vi "Autonomous Independent.vi"() -> ()   [LabVIEW 2016]
doc: "This VI is called when autonomous begins, and will automatically be terminated when autonomous ends. You can carry out timed or sensor driven robot movement independently without needing to return to the caller."
uses:
  <vilib>/Rock Robotics/WPI/ThirdParty/CanMotor/CTRLib-LV-TalonSRX/Framework/ServoParams.ctl
  <vilib>/Rock Robotics/WPI/ThirdParty/CanMotor/CTRLib-LV-TalonSRX/CTRE_CANTalonSRX_ControlMode.ctl
  <vilib>/Rock Robotics/WPI/Utilities/WPI_GetSetVariantRefNum.vi
  <vilib>/Rock Robotics/Network Tables/NT Write Numeric Array.vi
  <vilib>/Rock Robotics/WPI/ThirdParty/CanMotor/CTRLib-LV-TalonSRX/Framework/CTRE_ServoBlock_SmartTankStraightDistanceImu.vi
  <vilib>/Rock Robotics/WPI/ThirdParty/CanMotor/CTRLib-LV-TalonSRX/Framework/CTRE_ServoBlock_SmartTankTurnImu.vi
  <vilib>/Rock Robotics/WPI/ThirdParty/CanMotor/CTRLib-LV-TalonSRX/Framework/CTRE_ServoBlock_SmartTank.vi
panel:
  in  "Distance Params Back Up":T1={"P"=0.049999999999999996, "I"=0.001, "D"=0.017000000000000005, "I-Accum Max"=0.1, "I-Zone"=2.0, "Max Output"=0.5, "Nominal Output"=0.0, "Allowable Error"=0.0, "Reset I Accum"=FALSE}
  in  "Straight Params Back Up":T1={"P"=0.03, "I"=0.002, "D"=0.0, "I-Accum Max"=0.07, "I-Zone"=1.0, "Max Output"=0.15, "Nominal Output"=0.0, "Allowable Error"=0.5, "Reset I Accum"=FALSE}
  in  "Distance Params To Peg":T1={"P"=0.049999999999999996, "I"=0.001, "D"=0.017000000000000005, "I-Accum Max"=0.1, "I-Zone"=2.0, "Max Output"=0.5, "Nominal Output"=0.0, "Allowable Error"=0.0, "Reset I Accum"=FALSE}
  in  "Straight Params To Peg":T1={"P"=0.03, "I"=0.002, "D"=0.0, "I-Accum Max"=0.07, "I-Zone"=1.0, "Max Output"=0.15, "Nominal Output"=0.0, "Allowable Error"=0.5, "Reset I Accum"=FALSE}
  in  "Turn To Airship":T1={"P"=0.05, "I"=0.004, "D"=0.003, "I-Accum Max"=1.0, "I-Zone"=4.0, "Max Output"=0.2, "Nominal Output"=0.0, "Allowable Error"=0.0, "Reset I Accum"=FALSE}
  in  "Distance Params To Airship":T1={"P"=0.049999999999999996, "I"=0.001, "D"=0.017000000000000005, "I-Accum Max"=0.1, "I-Zone"=2.0, "Max Output"=0.5, "Nominal Output"=0.0, "Allowable Error"=0.0, "Reset I Accum"=FALSE}
  in  "Straight Params To Airship":T1={"P"=0.03, "I"=0.002, "D"=0.0, "I-Accum Max"=0.07, "I-Zone"=1.0, "Max Output"=0.15, "Nominal Output"=0.0, "Allowable Error"=0.5, "Reset I Accum"=FALSE}
  in  "Back Up\nFrom Peg":dbl=-20.0 format="%#_13g"
  in  "Angle\nTo Airship":dbl=30.0 format="%#_13g"
  in  "Distance\nTo Peg":dbl=55.0
  in  "Distance\nTo Airship":dbl=50.0
  # "Be sure to right-click and choose Data Operations>>Make Current Value default if you want to save the array values with the VI"
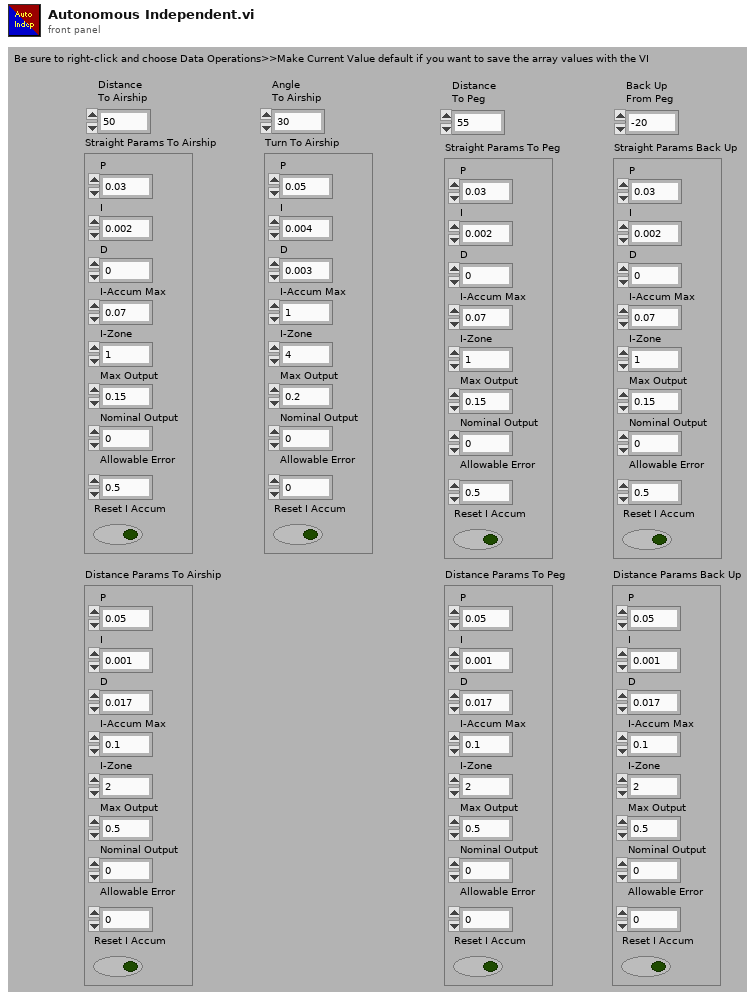
[diagram p1: front panel]
types:
  T1 = typedef "ServoParams.ctl" = cluster{"P":dbl, "I":dbl, "D":dbl, "I-Accum Max":dbl, "I-Zone":dbl, "Max Output":dbl, "Nominal Output":dbl, "Allowable Error":dbl, "Reset I Accum":bool}
  T2 = typedef "WPI_JoystickDevRef.ctl" = cluster{"Device":T3}
  T3 = typedef "WPI_JoystickDeviceEnum.ctl" = enum16{"USB 0", "USB 1", "USB 2", "USB 3", "USB 4", "USB 5"}
  T4 = typedef "SensoredTank.ctl" = cluster{"Sensored Gearbox Left":T5, "Sensored Gearbox Right ":T5, "Wheel Radius":dbl, "Distance Between Wheels":dbl}
  T5 = typedef "SensoredGearbox.ctl" = cluster{"Smart Motor Controller":T6, "Invert":bool, "Gear Ratio":dbl}
  T6 = typedef "WPI_MotorControlDeviceRef.ctl" = cluster{"DeviceStatus":errorcluster, "Type":T7, "PWM":cluster{"PWM Channel":T8, "DeadBand":T9}, "CAN":cluster{"Device Number":u8, "SetOutput VI Ref":variant, "GetOutput VI Ref":variant, "Enable VI Ref":variant, "Disable VI Ref":variant, "Data":variant}, "Invert":bool}
  T7 = typedef "WPI_MotorControlType.ctl" = enum16{"PWM", "CAN"}
  T8 = typedef "FPGA_DIOPWMChannel.ctl" = enum8{"PWM 0", "PWM 1", "PWM 2", "PWM 3", "PWM 4", "PWM 5", "PWM 6", "PWM 7", "PWM 8", "PWM 9", "PWM MXP 0", "PWM MXP 1", "PWM MXP 2", "PWM MXP 3", "PWM MXP 4", "PWM MXP 5", "PWM MXP 6", "PWM MXP 7", "PWM MXP 8", "PWM MXP 9", "Invalid"}
  T9 = typedef "WPI_PWMDeadband.ctl" = cluster{"Name":string, "maxPositivePwm":i32, "minPositivePwm":i32, "centerPwm":i32, "maxNegativePwm":i32, "minNegativePwm":i32, "angularRange":u16}
  T10 = typedef "CTRE_PigeonIMU_DeviceRef.ctl" = cluster{"DeviceStatus":errorcluster, "Device Number":u8, "Type":T11, "Device ID":u32, "Handle":u64, "UsageFrame":u32, "Library Path":path}
  T11 = typedef "CTRE_PigeonIMU_ConnectionType.ctl" = u32
  T12 = typedef "CTRE_CANTalonSRX_ControlMode.ctl" = enum16{"Throttle (Duty-Cycle)", "Position Closed-Loop", "Velocity Closed-Loop", "Current Closed-Loop", "Voltage Compensation", "Slave Follower", "Motion Profile", "Motion Magic"}
  T13 = cluster{"Sensored Tank":T4, "PigeonIMU":T10, "Talon SRX Control Mode":T12, "Set Heading":dbl, "Distance":dbl, "Distance Tolerance":dbl, "Straight Params":T1, "Distance Params":T1}
  T14 = cluster{"Servo Params":T1, "Sensored Tank":T4, "PigeonIMU":T10, "Talon SRX Control Mode":T12, "Angle Tolerance":dbl, "Set Angle":dbl}
  T15 = cluster{"Sensored Tank":T4, "Talon SRX Control Mode":T12, "Forward":dbl, "Turn":dbl}
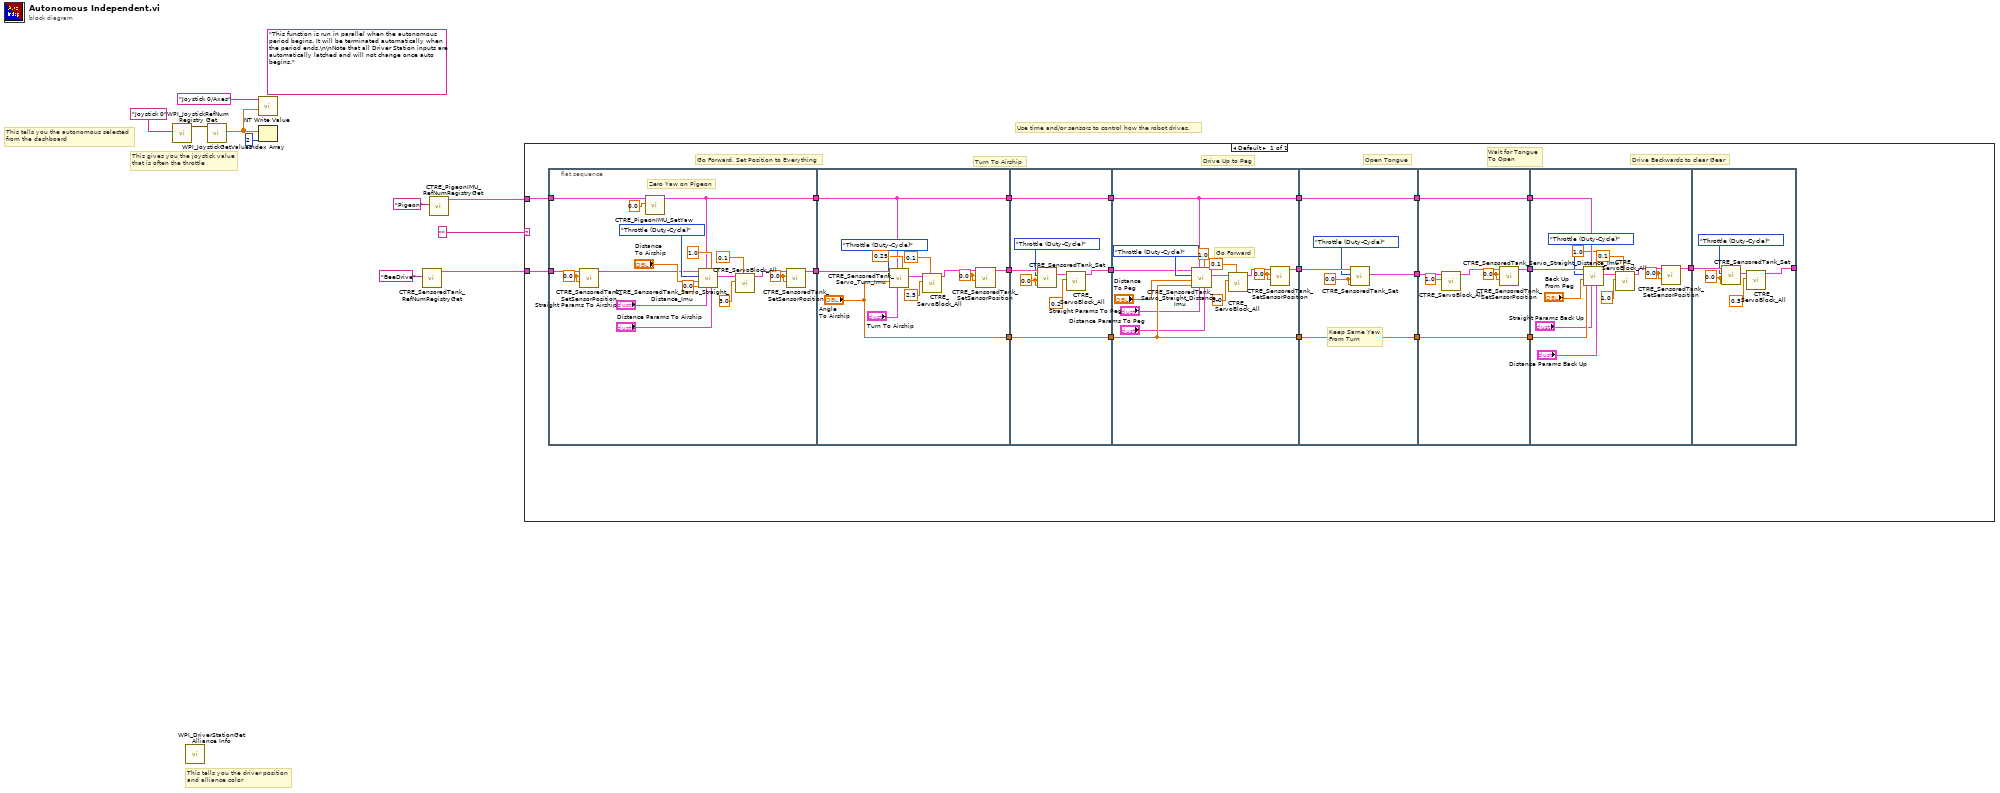
[diagram p0: block diagram]
diagram:
  (unwired) "This function is run in parallel when the autonomous period begins. It will be terminated automatically when the period ends.\n\nNote that all Driver Station inputs are automatically latched and will not change once auto begins."
  # "Use time and/or sensors to control how the robot drives."
  # "This tells you the autonomous selected\nfrom the dashboard"
  # "This gives you the joystick value\nthat is often the throttle"
  # "This tells you the driver position\nand alliance color"
  n1 = call <vilib>:"WPI_JoystickRefNum Registry Get.vi"("refnum name"="Joystick 0") -> ("JoystickDevRef"=w9:T2)  [unwired: 1 in, 9 out]
  n2 = call <vilib>:"WPI_DriverStationGet Alliance Info.vi"() -> ()  [unwired: 12 out]
  n3 = call <vilib>:"WPI_JoystickGetValues.vi"("JoystickDevRef"=w9) -> ("Axes"=w7:dbl[])  [unwired: 6 in, 4 out]
  n4 = call-poly <vilib>:"NT Write Value.vi"("Numeric Array"=w7, "Name"="Joystick 0/Axes") -> ()  [unwired: 9 in, 1 out]
  n5 = Index Array(array=w7, index=2) -> ()  [unwired: 1 out]
  n6 = call <vilib>:"CTRE_SensoredTank_RefNumRegistryGet.vi"("RefNum Name"="BeeDrive") -> ("Sensored Tank"=w3:T4)  [unwired: 10 in]
  n7 = call <vilib>:"CTRE_PigeonIMU_RefNumRegistryGet.vi"("refnum name"="Pigeon") -> ("PigeonIMUDevRef"=w1:T10)  [unwired: 9 in, 1 out]
  n8 = case shown="Default" "" {
    tunnel: w3 -> [w30]
    tunnel: w1 -> [w29]
    frame Default {
      # "Drive Backwards to clear Gear"
      # "Wait for Tongue\nTo Open"
      # "Open Tongue"
      # "Drive Up to Peg"
      # "Turn To Airship"
      # "Go Forward, Set Position to Everything"
      n9 = flat-sequence {
        tunnel: w30 -> [w35]
        tunnel: w29 -> [w44]
        tunnel: [w38] -> w28
        tunnel: [w40] -> w27
        tunnel: w28 -> [w60]
        tunnel: w27 -> [w55]
        tunnel: [w52] -> w16
        tunnel: [w55] -> w14
        tunnel: ["Angle\nTo Airship"] -> w12
        tunnel: w16 -> [w64]
        tunnel: [w63] -> w15
        tunnel: w14 -> [w68]
        tunnel: [w68] -> w13
        tunnel: w12 -> [w67]
        tunnel: [w67] -> w11
        tunnel: w15 -> [w77]
        tunnel: w13 -> [w76]
        tunnel: [w72] -> w26
        tunnel: [w76] -> w23
        tunnel: w11 -> [w75]
        tunnel: [w75] -> w18
        tunnel: w26 -> [w88]
        tunnel: [w85] -> w25
        tunnel: w23 -> [w84]
        tunnel: [w84] -> w22
        tunnel: [w83] -> w19
        tunnel: w18 -> [w83]
        tunnel: w25 -> [w95]
        tunnel: [w89] -> w24
        tunnel: w22 -> [w93]
        tunnel: [w93] -> w21
        tunnel: [w92] -> w20
        tunnel: w19 -> [w92]
        tunnel: w24 -> [w109]
        tunnel: w21 -> [w107]
        tunnel: w20 -> [w104]
        tunnel: [w99] -> w17
        tunnel: [w114] -> _
        tunnel: w17 -> [w112]
        frame #0 {
          w36 = 0.0 ("Left Side")
          w37 = 0.0 ("Left Side")
          # "Zero Yaw on Pigeon"
          n10 = call <vilib>:"CTRE_SensoredTank_SetSensorPosition.vi"("Right Side"=w36, "Left Side"=w36, "Sensored Tank"=w35) -> ("Sensored Tank"=w34:T4)  [unwired: 8 in]
          n11 = call <vilib>:"CTRE_PigeonIMU_SetYaw.vi"("Value"=0.0, "PigeonIMUDevRef"=w44) -> ("PigeonIMUDevRef"=w40:T10)  [unwired: 8 in, 1 out]
          n12 = call <vilib>:"CTRE_SensoredTank_Servo_Straight_Distance_Imu.vi"("Distance Params"="Distance Params To Airship", "Distance Tolerance"=1.0, "Straight Params"="Straight Params To Airship", "PigeonIMU"=w40, "Set Heading"=0.0, "Distance"="Distance\nTo Airship", "Talon SRX Control Mode"=CTRE_CANTalonSRX_ControlMode."Throttle (Duty-Cycle)", "Sensored Tank"=w34) -> ("Sensored Tank Distance IMU"=w42:T13)  [unwired: 1 in, 2 out]
          n13 = call-poly <vilib>:"CTRE_ServoBlock_All.vi"("Done Timeout"=0.1, "Timeout (s)"=3.0, "Sensored Tank Distance IMU"=w42) -> ("Sensored Tank"=w39:T4)  [unwired: 7 in, 1 out]
          n14 = call <vilib>:"CTRE_SensoredTank_SetSensorPosition.vi"("Right Side"=w37, "Left Side"=w37, "Sensored Tank"=w39) -> ("Sensored Tank"=w38:T4)  [unwired: 8 in]
        }
        frame #1 {
          w53 = 0.0 ("Left Side")
          n15 = call <vilib>:"CTRE_SensoredTank_Servo_Turn_Imu.vi"("Angle Tolerance"=0.25, "Servo Params"="Turn To Airship", "PigeonIMU"=w55, "Set Angle"="Angle\nTo Airship", "Talon SRX Control Mode"=CTRE_CANTalonSRX_ControlMode."Throttle (Duty-Cycle)", "Sensored Tank"=w60) -> ("Sensored Tank Servo Turn IMU"=w57:T14)  [unwired: 3 in, 2 out]
          n16 = call-poly <vilib>:"CTRE_ServoBlock_All.vi"("Done Timeout"=0.1, "Timeout (s)"=2.5, "Sensored Tank Servo Turn IMU"=w57) -> ("Sensored Tank"=w51:T4)  [unwired: 7 in, 1 out]
          n17 = call <vilib>:"CTRE_SensoredTank_SetSensorPosition.vi"("Right Side"=w53, "Left Side"=w53, "Sensored Tank"=w51) -> ("Sensored Tank"=w52:T4)  [unwired: 8 in]
        }
        frame #2 {
          w61 = 0.0 ("Forward")
          n18 = call <vilib>:"CTRE_SensoredTank_Set.vi"("Turn"=w61, "Forward"=w61, "Talon SRX Control Mode"=CTRE_CANTalonSRX_ControlMode."Throttle (Duty-Cycle)", "Sensored Tank"=w64) -> ("SmartTank"=w66:T15)  [unwired: 6 in, 1 out]
          n19 = call-poly <vilib>:"CTRE_ServoBlock_All.vi"("Timeout"=0.2, "SmartTank"=w66) -> ("Sensored Tank"=w63:T4)  [unwired: 9 in]
        }
        frame #3 {
          w74 = 0.0 ("Left Side")
          # "Go Forward"
          n20 = call <vilib>:"CTRE_SensoredTank_Servo_Straight_Distance_Imu.vi"("Distance Params"="Distance Params To Peg", "Distance Tolerance"=1.0, "Straight Params"="Straight Params To Peg", "PigeonIMU"=w76, "Set Heading"=w75, "Distance"="Distance\nTo Peg", "Talon SRX Control Mode"=CTRE_CANTalonSRX_ControlMode."Throttle (Duty-Cycle)", "Sensored Tank"=w77) -> ("Sensored Tank Distance IMU"=w79:T13)  [unwired: 1 in, 2 out]
          n21 = call-poly <vilib>:"CTRE_ServoBlock_All.vi"("Done Timeout"=0.1, "Timeout (s)"=3.0, "Sensored Tank Distance IMU"=w79) -> ("Sensored Tank"=w73:T4)  [unwired: 7 in, 1 out]
          n22 = call <vilib>:"CTRE_SensoredTank_SetSensorPosition.vi"("Right Side"=w74, "Left Side"=w74, "Sensored Tank"=w73) -> ("Sensored Tank"=w72:T4)  [unwired: 8 in]
        }
        frame #4 {
          w86 = 0.0 ("Forward")
          # "Keep Same Yaw \nFrom Turn"
          n23 = call <vilib>:"CTRE_SensoredTank_Set.vi"("Turn"=w86, "Forward"=w86, "Talon SRX Control Mode"=CTRE_CANTalonSRX_ControlMode."Throttle (Duty-Cycle)", "Sensored Tank"=w88) -> ("SmartTank"=w85:T15)  [unwired: 6 in, 1 out]
        }
        frame #5 {
          w91 = 0.0 ("Left Side")
          n24 = call-poly <vilib>:"CTRE_ServoBlock_All.vi"("Timeout"=1.0, "SmartTank"=w95) -> ("Sensored Tank"=w90:T4)  [unwired: 9 in]
          n25 = call <vilib>:"CTRE_SensoredTank_SetSensorPosition.vi"("Right Side"=w91, "Left Side"=w91, "Sensored Tank"=w90) -> ("Sensored Tank"=w89:T4)  [unwired: 8 in]
        }
        frame #6 {
          w101 = 0.0 ("Left Side")
          n26 = call <vilib>:"CTRE_SensoredTank_Servo_Straight_Distance_Imu.vi"("Distance Params"="Distance Params Back Up", "Distance Tolerance"=1.0, "Straight Params"="Straight Params Back Up", "PigeonIMU"=w107, "Set Heading"=w104, "Distance"="Back Up\nFrom Peg", "Talon SRX Control Mode"=CTRE_CANTalonSRX_ControlMode."Throttle (Duty-Cycle)", "Sensored Tank"=w109) -> ("Sensored Tank Distance IMU"=w103:T13)  [unwired: 1 in, 2 out]
          n27 = call-poly <vilib>:"CTRE_ServoBlock_All.vi"("Done Timeout"=0.1, "Timeout (s)"=1.0, "Sensored Tank Distance IMU"=w103) -> ("Sensored Tank"=w100:T4)  [unwired: 7 in, 1 out]
          n28 = call <vilib>:"CTRE_SensoredTank_SetSensorPosition.vi"("Right Side"=w101, "Left Side"=w101, "Sensored Tank"=w100) -> ("Sensored Tank"=w99:T4)  [unwired: 8 in]
        }
        frame #7 {
          w113 = 0.0 ("Forward")
          n29 = call <vilib>:"CTRE_SensoredTank_Set.vi"("Turn"=w113, "Forward"=w113, "Talon SRX Control Mode"=CTRE_CANTalonSRX_ControlMode."Throttle (Duty-Cycle)", "Sensored Tank"=w112) -> ("SmartTank"=w111:T15)  [unwired: 6 in, 1 out]
          n30 = call-poly <vilib>:"CTRE_ServoBlock_All.vi"("Timeout"=0.5, "SmartTank"=w111) -> ("Sensored Tank"=w114:T4)  [unwired: 9 in]
        }
      }
    }
  }
